vi "main splash.vi"() -> ()   [LabVIEW 2013, in "Standard Editor.lvlib" / "splash screen.lvlib"]
uses:
  splash screen.lvlib
  notifier data.ctl
panel:
  in  "notifier":refnum<notifier>
  in  "stop":bool
  in  "error in":errorcluster
  out "Progress":dbl(slide) scale=0.0..100.0
  out "Text":string
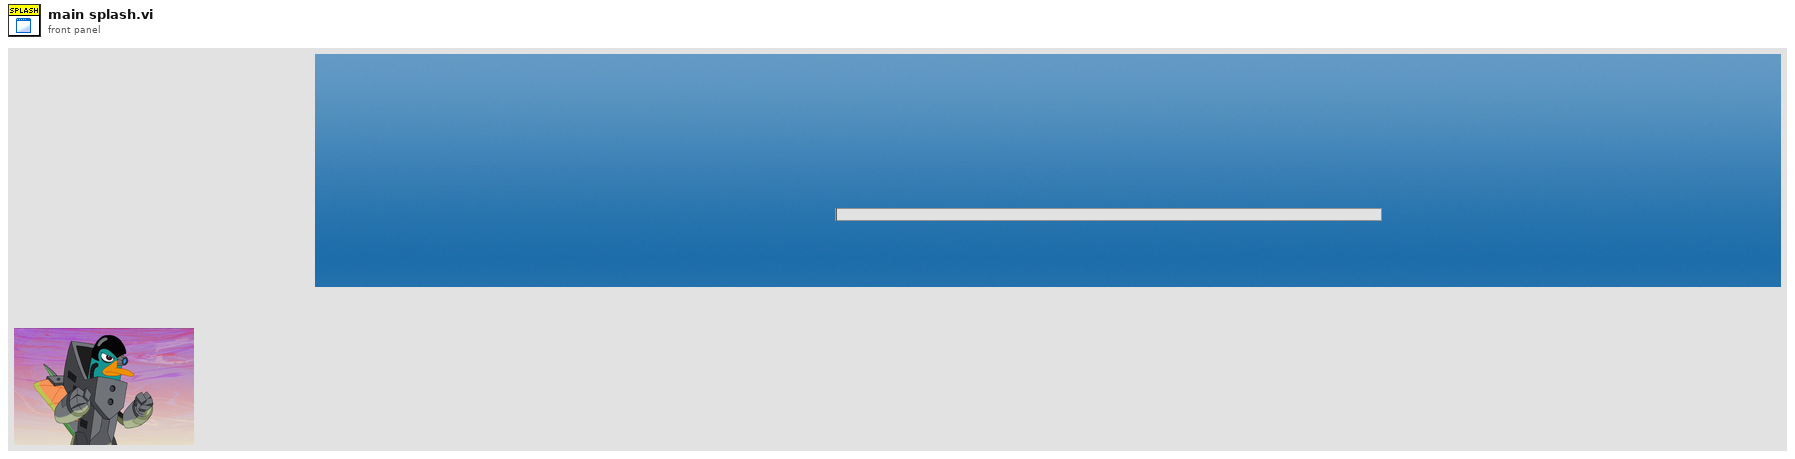
[diagram p1: front panel]
types:
  T1 = typedef "Standard Editor.lvlib/splash screen.lvlib/notifier data.ctl" = cluster{"Text":string, "percent":dbl}
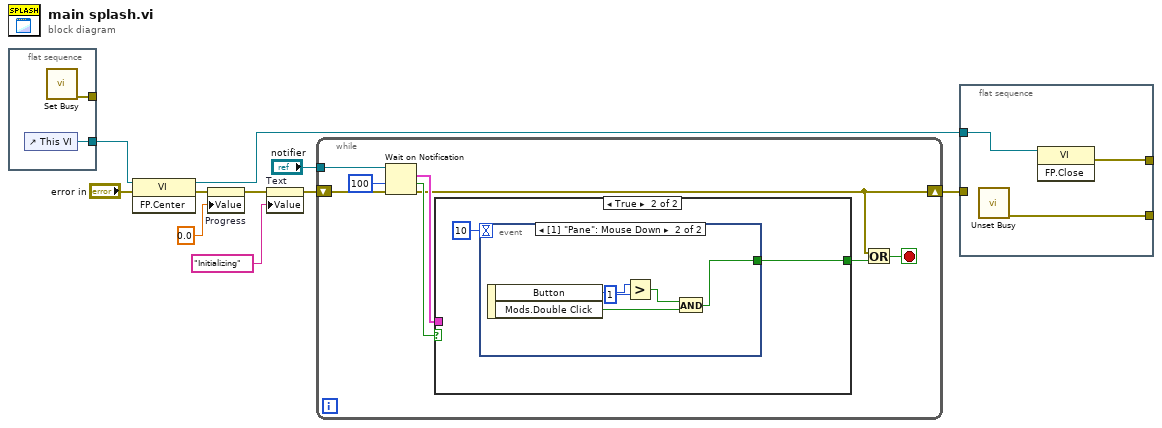
[diagram p0: block diagram]
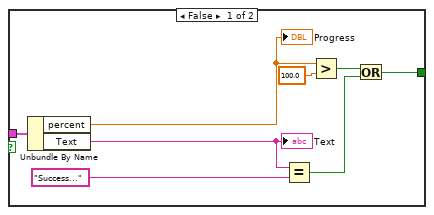
[diagram p2: hidden frame]
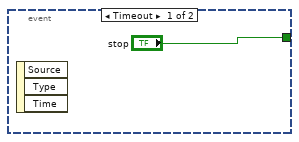
[diagram p3: hidden frame]
diagram:
  n1 = flat-sequence {
    tunnel: [w12] -> w6
    tunnel: [w11] -> _
    frame #0 {
      n2 = control-ref of="This VI"() -> (w12:refnum<vi>)
      n3 = call <vilib>:"Set Busy.vi"() -> ("error out"=w11:errorcluster)  [unwired: 10 in, 1 out]
    }
  }
  n4 = invoke class="VI" method="FP.Center"(reference=w6, error in="error in") -> (reference out=w1:refnum<vi>, error out=w4:errorcluster)  [unwired: 1 in, 1 out]
  n5 = property on="Progress" class="Slide (strict)"(error in=w4, "Value"=0.0 ("Progress")) -> (error out=w8:errorcluster)  [unwired: 1 in, 1 out]
  n6 = property on="Text" class="Str"(error in=w8, "Value"="Initializing" ("Text")) -> (error out=w10:errorcluster)  [unwired: 1 in, 1 out]
  n7 = while {
    tunnel: "notifier" -> [w20]
    shift-right: [w13] -> w2
    shift-left: w10 -> [w17]
    stop <- w14 stop-if-true
    n8 = Wait on Notification(notifier=w20, timeout in ms (-1)=100, error in (no error)=w17) -> (notification=w18:T1, timed out?=w19:bool, error out=w13:errorcluster)  [unwired: 1 in, 1 out]
    n9 = case shown="True" w19 {
      tunnel: [w24 w29] -> w16
      tunnel: w18 -> [w28 _]
      frame False {
        n10 = Unbundle By Name(w28) -> ("percent"=w23:dbl, "Text"=w25:string)
        "Text" <- w25
        "Progress" <- w23
        n11 = Equal?(x=w25, y="Success...") -> (x = y?=w26:bool)
        n12 = Greater?(x=w23, y=100.0) -> (0:w21:bool)
        n13 = Or(x=w21, y=w26) -> (x .or. y?=w24:bool)
      }
      frame True {
        n14 = event shown="[1] \"Pane\": Mouse Down" {
          selector: _ -> [_ _]
          dyn-events: _ -> [_ _]
          timeout: 10 -> [_ _]
          tunnel: ["stop" w32] -> w29
          event Timeout {
            n15 = event-data() -> ()  [unwired: 1 in, 3 out]
          }
          event Mouse Down {
            n16 = event-data() -> ("Button"=w35:u16, "Mods.Double Click"=w36:bool)  [unwired: 1 in]
            n17 = Greater?(x=w35, y=u16 1) -> (0:w33:bool)
            n18 = And(x=w33, y=w36) -> (x .and. y?=w32:bool)
          }
        }
      }
    }
    n19 = Or(x=w13, y=w16) -> (x .or. y?=w14:bool)
  }
  n20 = flat-sequence {
    tunnel: [w39] -> _
    tunnel: w2 -> [_]
    tunnel: w1 -> [w38]
    tunnel: [w37] -> _
    frame #0 {
      n21 = call <vilib>:"Unset Busy.vi"() -> ("error out"=w39:errorcluster)  [unwired: 11 in]
      n22 = invoke class="VI" method="FP.Close"(reference=w38) -> (error out=w37:errorcluster)  [unwired: 2 in, 2 out]
    }
  }
